vi "Script_Timing_Replace_Template_Values.vi"(8 "error in (no error)":errorcluster, 10 "Mandatory Items":T2={"Script Name"="Template_For%ions + 50 repeats", "GINI Time Period"=100000.0, "HSDIO Delay"=30.0, "Shutter Duration before"=50000.0, "Shutter Duration after"=50000.0, "Filter Tau"=2000.0, "Emtyping Duration"=1000000.0} caption="TIMING Mandatory Items" {"GINI Time Period" min=100000.0 max=1000000.0 format="%#_7g"; "Shutter Duration after" min=2.0 max=100000.0; "HSDIO Delay" min=0.0 max=100.0; "Shutter Duration before" min=2.0 max=100000.0; "Filter Tau" min=1000.0 max=2000.0; "Emtyping Duration" min=2.0 format="%#_8g"}) -> (0 "error out":errorcluster, 3 "Ouput Script":string)   [LabVIEW 2018]
doc: "This VI replaces the macros strings of the template timing script by the TIMING Mandatory tems."
uses:
  controls/TIMING_Mandatory_Items.ctl
  controls/TRAPPING_Inputs.ctl
  controls/EXPERT_Path_Selector.ctl
panel:
  in  "TRAPPING Inputs":T1={"Number of Channels"=4, "Init Values"=[2.0, 9.0, 2.0, 9.0], "Opening Values"=[0.0, 0.0, 0.0, 0.0], "Trapping Values"=[2.0, 9.0, 2.0, 9.0], "Emptying Values"=[-10.0, -10.0, -10.0, -10.0], "Adiabatic ON"=FALSE, "Adiabatic Duration"=100, "Adiabatic Waveforms"=["Adiabatic_None_2_2_2000", "Adiabatic_Ramp_9_0_2000", "Adiabatic_None_2_2_2000", "Adiabatic_RC_9_0_2000"], "Ions Refill ON"=FALSE, "Number of Ions Refills"=1, "Trapping Delay"=400.0, "Trapping Duration"=300.0} {"Trapping Duration" min=2.0; "Trapping Delay" min=2.0; "Number of Ions Refills" min=1 max=1000; "Trapping Values" min=-10.0 max=10.0; "Init Values" min=-10.0 max=10.0; "Emptying Values" min=-10.0 max=10.0; "Opening Values" min=-10.0 max=10.0}
  # "GO_out"
  # "Gout"
  # "GI_in"
  # "Gin"
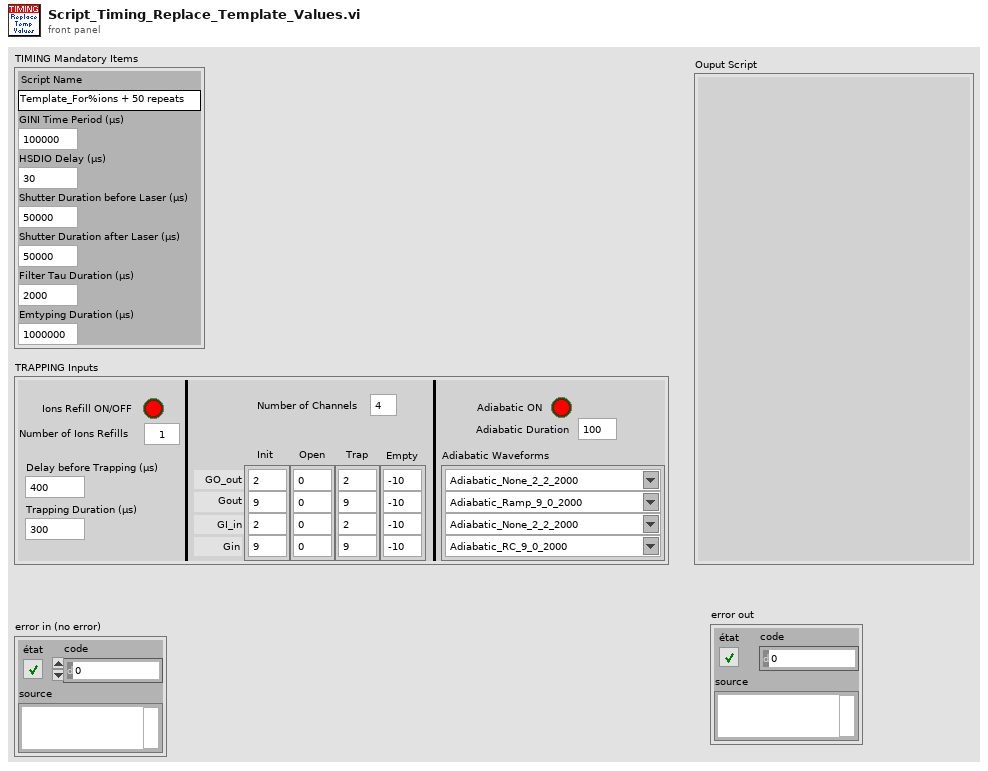
[diagram p1: front panel]
types:
  T1 = typedef "TRAPPING_Inputs.ctl" = cluster{"Number of Channels":i32, "Init Values":dbl[], "Opening Values":dbl[], "Trapping Values":dbl[], "Emptying Values":dbl[], "Adiabatic ON":bool, "Adiabatic Duration":i32, "Adiabatic Waveforms":string[], "Ions Refill ON":bool, "Number of Ions Refills":i32, "Trapping Delay":dbl, "Trapping Duration":dbl}
  T2 = typedef "TIMING_Mandatory_Items.ctl" = cluster{"Script Name":string, "GINI Time Period":dbl, "HSDIO Delay":dbl, "Shutter Duration before":dbl, "Shutter Duration after":dbl, "Filter Tau":dbl, "Emtyping Duration":dbl}
  T3 = typedef "EXPERT_Path_Selector.ctl" = enum16{"Application", "Resources", "Data", "XML", "XML Saved", "Load Directory"}
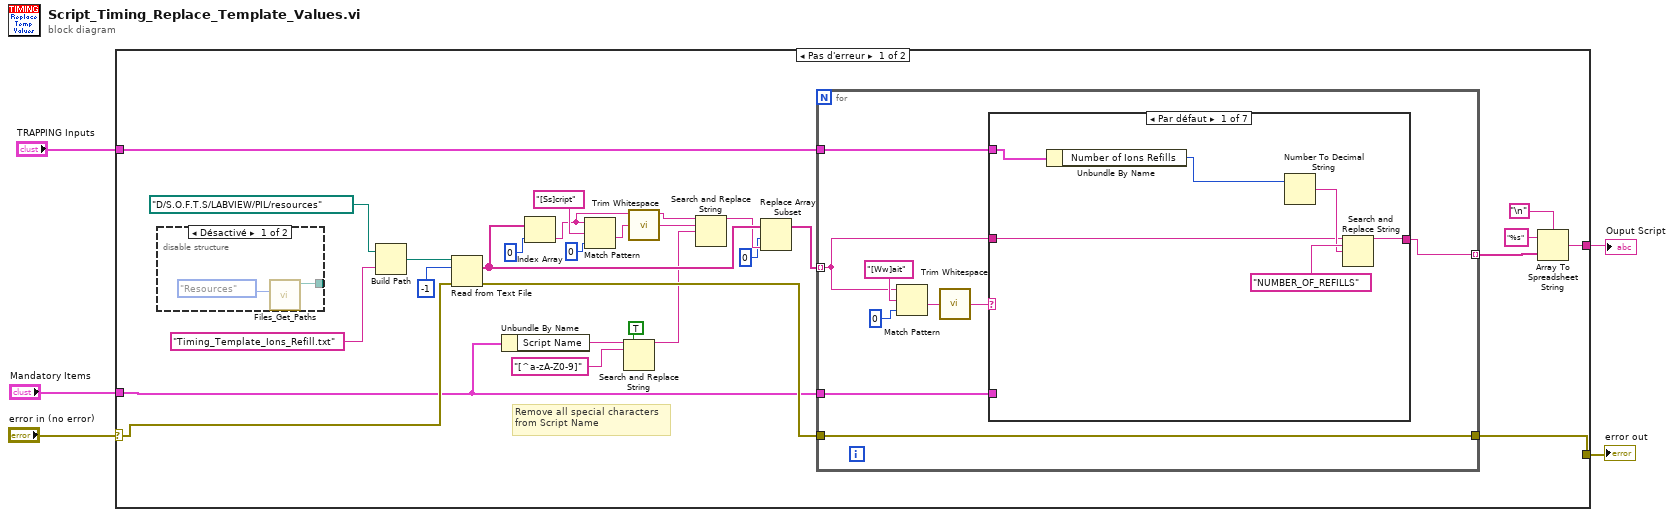
[diagram p0: block diagram]
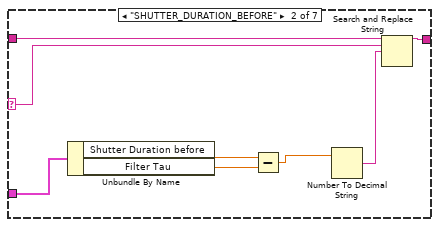
[diagram p3: hidden frame]
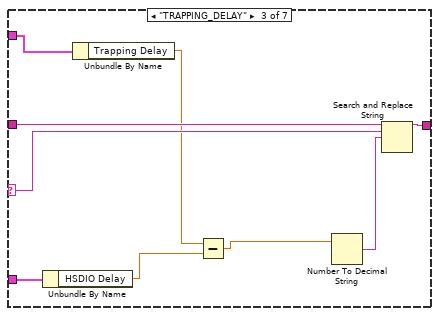
[diagram p4: hidden frame]
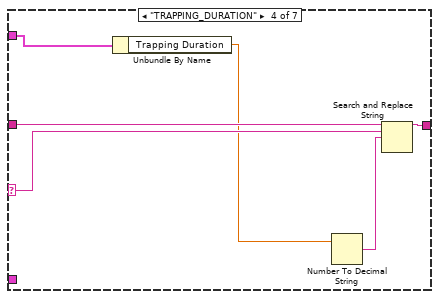
[diagram p5: hidden frame]
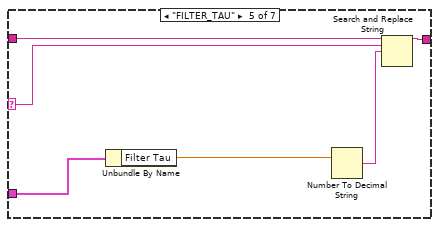
[diagram p6: hidden frame]
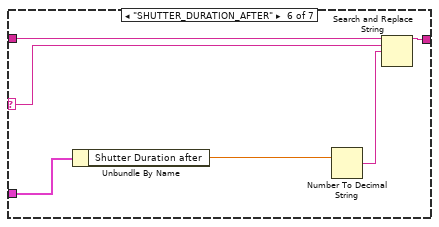
[diagram p7: hidden frame]
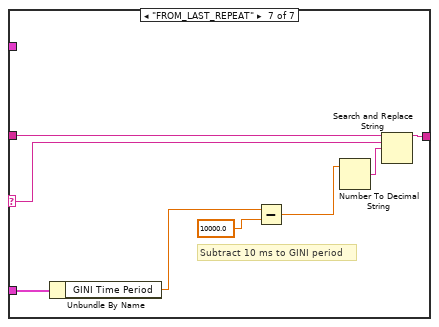
[diagram p8: hidden frame]
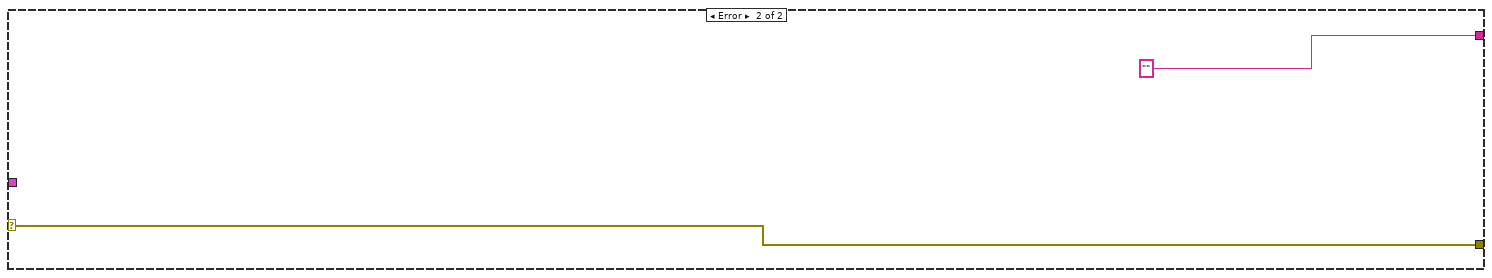
[diagram p9: hidden frame]
diagram:
  n1 = case shown="Pas d'erreur" "error in (no error)" {
    selector: "error in (no error)" -> [w29 w94]
    tunnel: [w28 w94] -> w4
    tunnel: "Mandatory Items" -> [w6 _]
    tunnel: [w24 "" ("spreadsheet string")] -> w2
    tunnel: "TRAPPING Inputs" -> [w11 _]
    frame No Error {
      # "Remove all special characters\nfrom Script Name"
      n2 = disable-structure shown="Désactivé" {
        disable-tunnel: [w33 _] -> _
        frame Disabled {
          n3 = call "Files_Get_Paths.vi"("EXPERT Path Selector"=EXPERT_Path_Selector."Resources") -> ("Path"=w33:path)  [unwired: 9 in, 1 out]
        }
        frame Enabled {
        }
      }
      n4 = Build Path(base path=path "D:/S.O.F.T.S/LABVIEW/PIL/resources" ("Path"), name or relative path="Timing_Template_Ions_Refill.txt" ("nom ou chemin relatif")) -> (appended path=w31:path)
      n5 = Read from Text File(file (use dialog)=w31, count=-1 ("nombre"), error in=w29) -> (text=w16:string[], error out=w27:errorcluster)  [unwired: 1 in, 2 out]
      n6 = Unbundle By Name(w6) -> ("Script Name"=w8:string)
      n7 = Index Array(array=w16, index=0 ("indice")) -> (element=w17:string)
      n8 = Match Pattern(string=w17, regular expression="[Ss]cript" ("expression régulière"), offset (0)=0) -> (after substring=w19:string)  [unwired: 3 out]
      n9 = Search and Replace String(replace all?=TRUE ("tout remplacer ? (F)"), input string=w8, search string="[^a-zA-Z0-9]" ("expression régulière")) -> (result string=w7:string)  [unwired: 5 in, 3 out]
      n10 = call <vilib>:"Trim Whitespace.vi"("string"=w19) -> ("trimmed string"=w18:string)  [unwired: 1 in]
      n11 = Search and Replace String(input string=w17, search string=w18, replace string=w7) -> (result string=w15:string)  [unwired: 5 in, 3 out]
      n12 = Replace Array Subset(array=w16, new element=w15, index=0 ("indice")) -> (w13:string[])
      n13 = for {
        tunnel: w27 -> [w41]
        tunnel: [w41] -> w28
        tunnel: w6 -> [w39]
        tunnel: [w37] -> w26 mode=indexing
        tunnel: w13 -> [w36] mode=indexing
        tunnel: w11 -> [w35]
        n14 = Match Pattern(string=w36, regular expression="[Ww]ait", offset (0)=0) -> (after substring=w42:string)  [unwired: 3 out]
        n15 = call <vilib>:"Trim Whitespace.vi"("string"=w42) -> ("trimmed string"=w40:string)  [unwired: 1 in]
        n16 = case shown="Par défaut" w40 {
          selector: w40 -> [_ w56 w66 w72 w77 w83 w92]
          tunnel: w39 -> [_ w57 w60 _ w78 w84 w86]
          tunnel: [w47 w55 w65 w71 w76 w82 w91] -> w37
          tunnel: w36 -> [w46 w50 w63 w69 w73 w79 w89]
          tunnel: w35 -> [w45 _ w62 w68 _ _ _]
          frame Default {
            n17 = Unbundle By Name(w45) -> ("Number of Ions Refills"=w44:i32)
            n18 = Number To Decimal String(number=w44) -> (decimal integer string=w48:string)  [unwired: 1 in]
            n19 = Search and Replace String(input string=w46, search string="NUMBER_OF_REFILLS" ("chaîne recherchée"), replace string=w48) -> (result string=w47:string)  [unwired: 5 in, 3 out]
          }
          frame "SHUTTER_DURATION_BEFORE" {
            n20 = Unbundle By Name(w57) -> ("Shutter Duration before"=w53:dbl, "Filter Tau"=w52:dbl)
            n21 = Subtract(x=w53, y=w52) -> (x-y=w51:dbl)
            n22 = Number To Decimal String(number=w51) -> (decimal integer string=w54:string)  [unwired: 1 in]
            n23 = Search and Replace String(input string=w50, search string=w56, replace string=w54) -> (result string=w55:string)  [unwired: 5 in, 3 out]
          }
          frame "TRAPPING_DELAY" {
            n24 = Unbundle By Name(w60) -> ("HSDIO Delay"=w58:dbl)
            n25 = Unbundle By Name(w62) -> ("Trapping Delay"=w61:dbl)
            n26 = Subtract(x=w61, y=w58) -> (x-y=w59:dbl)
            n27 = Number To Decimal String(number=w59) -> (decimal integer string=w64:string)  [unwired: 1 in]
            n28 = Search and Replace String(input string=w63, search string=w66, replace string=w64) -> (result string=w65:string)  [unwired: 5 in, 3 out]
          }
          frame "TRAPPING_DURATION" {
            n29 = Unbundle By Name(w68) -> ("Trapping Duration"=w67:dbl)
            n30 = Number To Decimal String(number=w67) -> (decimal integer string=w70:string)  [unwired: 1 in]
            n31 = Search and Replace String(input string=w69, search string=w72, replace string=w70) -> (result string=w71:string)  [unwired: 5 in, 3 out]
          }
          frame "FILTER_TAU" {
            n32 = Unbundle By Name(w78) -> ("Filter Tau"=w74:dbl)
            n33 = Number To Decimal String(number=w74) -> (decimal integer string=w75:string)  [unwired: 1 in]
            n34 = Search and Replace String(input string=w73, search string=w77, replace string=w75) -> (result string=w76:string)  [unwired: 5 in, 3 out]
          }
          frame "SHUTTER_DURATION_AFTER" {
            n35 = Unbundle By Name(w84) -> ("Shutter Duration after"=w80:dbl)
            n36 = Number To Decimal String(number=w80) -> (decimal integer string=w81:string)  [unwired: 1 in]
            n37 = Search and Replace String(input string=w79, search string=w83, replace string=w81) -> (result string=w82:string)  [unwired: 5 in, 3 out]
          }
          frame "FROM_LAST_REPEAT" {
            # "Subtract 10 ms to GINI period"
            n38 = Unbundle By Name(w86) -> ("GINI Time Period"=w85:dbl)
            n39 = Subtract(x=w85, y=10000.0) -> (x-y=w87:dbl)
            n40 = Number To Decimal String(number=w87) -> (decimal integer string=w90:string)  [unwired: 1 in]
            n41 = Search and Replace String(input string=w89, search string=w92, replace string=w90) -> (result string=w91:string)  [unwired: 5 in, 3 out]
          }
        }
      }
      n42 = Array To Spreadsheet String(delimiter (Tab)="\n", array=w26, 3:"%s" ("chaîne de format")) -> (spreadsheet string=w24:string)
    }
    frame Error {
    }
  }
  "error out" <- w4
  "Ouput Script" <- w2
